vi "OOP SM.vi"   [LabVIEW 2020, in "OOP SM.lvlib"]
uses:
  OOP SM.lvlib
  Message/Message.lvclass
  Init Msg/Init Msg.lvclass
  E:/NI I Program/Actor Intr Demo/OOP SM/Message/Message.lvclass
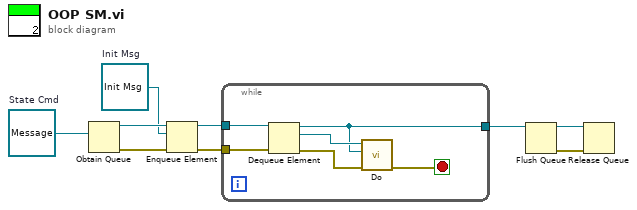
[diagram p0: block diagram]
diagram:
  w7 = refnum<class "Init Msg.lvclass"> refnum  # Init Msg
  w9 = refnum<class "Message.lvclass"> refnum  # State Cmd
  n1 = Obtain Queue(element data type=w9) -> (queue out=w8:refnum<queue>, error out=w6:errorcluster)  [unwired: 4 in, 1 out]
  n2 = Enqueue Element(queue=w8, element=w7, error in (no error)=w6) -> (queue out=w5:refnum<queue>, error out=w4:errorcluster)  [unwired: 1 in, 1 out]
  n3 = while {
    tunnel: w5 -> [w15]
    tunnel: w4 -> [w14]
    tunnel: [w10] -> w3
    stop <- w11 stop-if-true
    n4 = Dequeue Element(queue=w15, error in (no error)=w14) -> (queue out=w10:refnum<queue>, element=w13:refnum<class "Message.lvclass">, error out=w12:errorcluster)  [unwired: 1 in, 1 out]
    n5 = call-dynamic "Do.vi"("error in (no error)"=w12, "queue out"=w10, "State Cmd in"=w13) -> ("error out"=w11:errorcluster)  [unwired: 7 in, 1 out]
  }
  n6 = Flush Queue(queue=w3) -> (queue out=w2:refnum<queue>, error out=w1:errorcluster)  [unwired: 1 in, 1 out]
  n7 = Release Queue(queue=w2, error in (no error)=w1) -> ()  [unwired: 1 in, 3 out]
